vi "Get Property.vi"(10 "Ctl Ref":refnum<vi>, 11 "UIP In":refnum<class "UIP.lvclass">) -> (0 "Error Out":errorcluster, 3 "UIP Out":refnum<class "UIP.lvclass">)   [LabVIEW 2015, in "UIP.lvclass"]
doc: "Overwrite this abstract method to implement child behavior for getting the property from the VI Server Control and into the UIP private data."
uses:
  UIP.lvclass
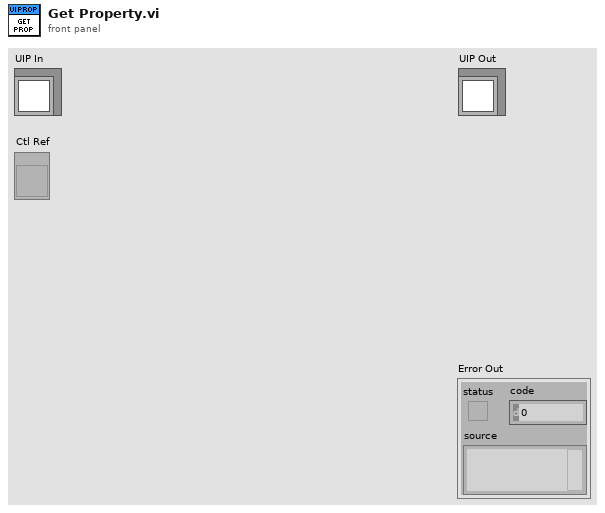
[diagram p1: front panel]
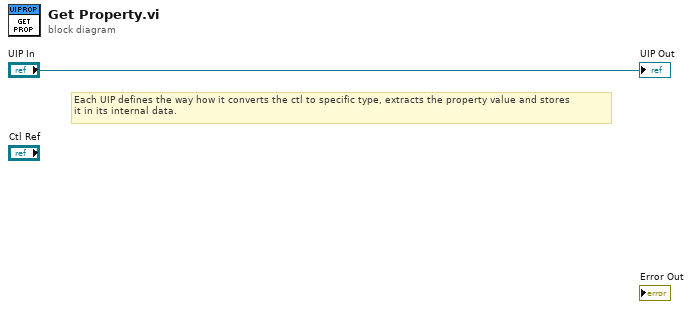
[diagram p0: block diagram]
diagram:
  # "Each UIP defines the way how it converts the ctl to specific type, extracts the property value and stores\nit in its internal data."
  "UIP Out" <- "UIP In"
